vi "SaveCameraSettings.vi"(0 "object in":refnum<class "Experiment2.lvclass">, 1 "ReadoutTime":dbl, 2 "Sub Region":T1 {"V Size"."Value" min=0 max=0 step=4; "H Size"."Value" min=0 max=0 step=4; "V Offset"."Value" min=0 max=0 step=4; "H Offset"."Value" min=0 max=0 step=4}, 5 "error in (no error)":errorcluster) -> (14 "object out":refnum<class "Experiment2.lvclass">, 19 "error out":errorcluster)   [LabVIEW 2024, in "Experiment2.lvclass"]
uses:
  Experiment2.lvclass
  Hamamatsu_class/SubRegionLimits.ctl
  <vilib>/Utility/miscctls.llb/LVMinMaxIncTypeDef.ctl
  Experiment2.lvclass/Experiment2.ctl
  Hamamatsu_class/Hamamatsu.lvclass
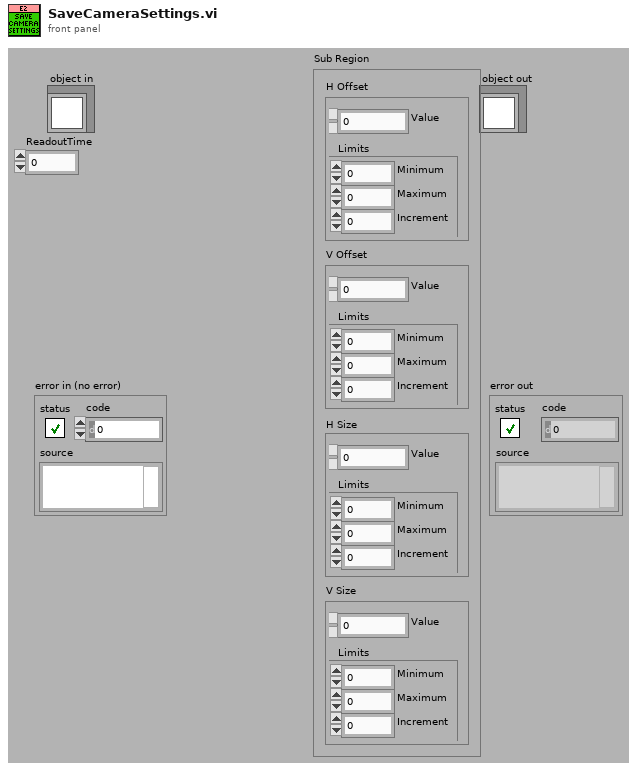
[diagram p1: front panel]
types:
  T1 = typedef "Hamamatsu.lvclass/SubRegionLimits.ctl" = cluster{"H Offset":cluster{"Value":i32, "Limits":T2}, "V Offset":cluster{"Value":i32, "Limits":T2}, "H Size":cluster{"Value":i32, "Limits":T2}, "V Size":cluster{"Value":i32, "Limits":T2}}
  T2 = typedef "LVMinMaxIncTypeDef.ctl" = cluster{"Minimum":dbl, "Maximum":dbl, "Increment":dbl}
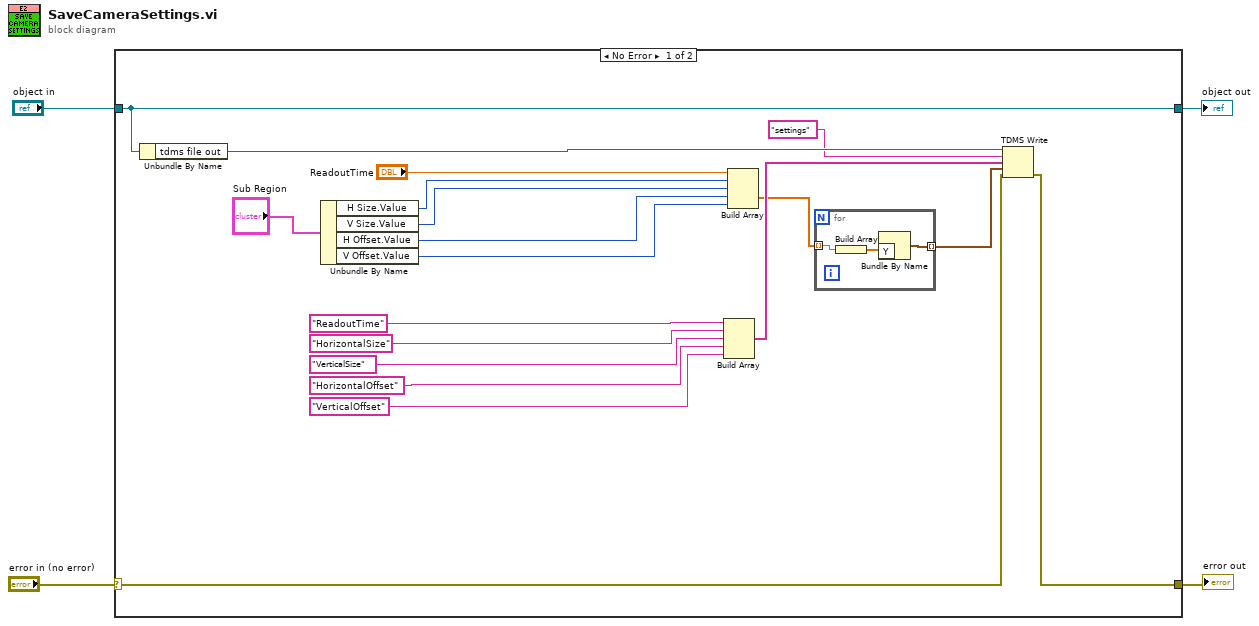
[diagram p0: block diagram]
diagram:
  n1 = case shown="No Error" "error in (no error)" {
    selector: "error in (no error)" -> [w21 w28]
    tunnel: [w16 w28] -> w3
    tunnel: [w23 w27] -> w1
    tunnel: "object in" -> [w23 w27]
    frame No Error {
      n2 = Unbundle By Name(w23) -> ("tdms file out"=w22:refnum<k34>)
      n3 = Unbundle By Name("Sub Region") -> ("H Size.Value"=w8:i32, "V Size.Value"=w7:i32, "H Offset.Value"=w6:i32, "V Offset.Value"=w5:i32)
      n4 = Build Array("ReadoutTime", "HorizontalSize", "VerticalSize", "HorizontalOffset", "VerticalOffset") -> (w20:string[])
      n5 = Build Array("ReadoutTime", w8, w7, w6, w5) -> (w19:dbl[])
      n6 = for {
        tunnel: w19 -> [w26] mode=indexing
        tunnel: [w24] -> w18 mode=indexing
        n7 = Build Array(w26) -> (w25:dbl[])
        n8 = Bundle By Name("Y"=w25) -> (w24:waveform(dbl))  [unwired: 1 in]
      }
      n9 = TDMS Write(0:w22, 5:"settings" ("group name in (Untitled)"), 7:w20, 9:w18, 11:w21) -> (15:w16:errorcluster)  [unwired: 1 in, 3 out]
    }
    frame Error {
    }
  }
  "error out" <- w3
  "object out" <- w1
